vi "Init MCListbox Color.vi"(0 "Array of Checks":bool[](array[boolean]), 1 "Cols indices to set color":u8[](array[numeric]), 2 "Multicolumn Listbox Ref":refnum<vi>) -> ()   [LabVIEW 2016, in "TSPopup.lvlib"]
uses:
  <userlib>/TSPopup/TSPopup.lvlib
  <vilib>/Utility/miscctls.llb/LVRowAndColumnTypeDef.ctl
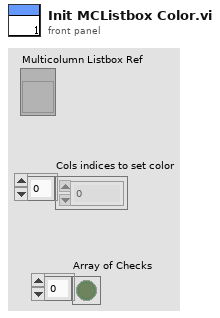
[diagram p1: front panel]
types:
  T1 = typedef "LVRowAndColumnTypeDef.ctl" = cluster{"Row":i32, "Column":i32}
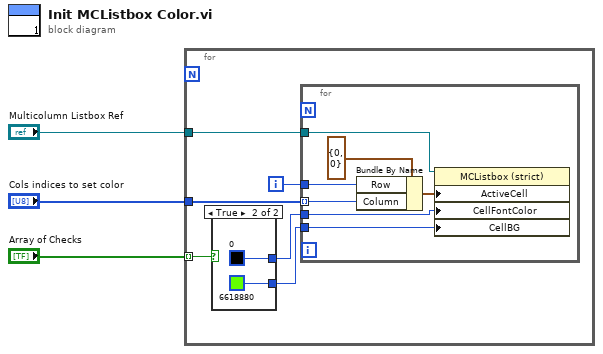
[diagram p0: block diagram]
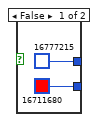
[diagram p2: hidden frame]
diagram:
  n1 = for {
    tunnel: "Array of Checks" -> [w8] mode=indexing
    tunnel: "Multicolumn Listbox Ref" -> [w9]
    tunnel: "Cols indices to set color" -> [w6]
    i -> [w7]
    n2 = case shown="True" w8 {
      tunnel: [u32 16711680 u32 6618880] -> w4
      tunnel: [u32 16777215 u32 0] -> w5
      frame False {
      }
      frame True {
      }
    }
    n3 = for {
      tunnel: w9 -> [w16]
      tunnel: w7 -> [w13]
      tunnel: w6 -> [w12] mode=indexing
      tunnel: w5 -> [w11]
      tunnel: w4 -> [w10]
      n4 = Bundle By Name(cluster=T1 {"Row"=0, "Column"=0} ("Active Cell:Active Cell"), "Row"=w13, "Column"=w12) -> (w14:T1)
      n5 = property class="MCListbox (strict)"(reference=w16, "ActiveCell"=w14, "CellFontColor"=w11, "CellBG"=w10) -> ()  [unwired: 1 in, 2 out]
    }
  }
